vi "MatrixMult (SubVI).vi"(0 "I":fxp<+/-,32,16>, 1 "1,1":fxp<+/-,32,16>, 2 "1, 2":fxp<+/-,32,16>, 3 "1, 3":fxp<+/-,32,16>, 5 "x":fxp<+/-,32,16>, 7 "y":fxp<+/-,32,16>, 9 "3, 1":fxp<+/-,32,16>, 10 "3, 3":fxp<+/-,32,16>, 11 "3, 2":fxp<+/-,32,16>, 12 "2, 1":fxp<+/-,32,16>, 13 "2, 2":fxp<+/-,32,16>, 14 "2, 3":fxp<+/-,32,16>) -> (4 "v1":fxp<+/-,32,16>, 6 "v2":fxp<+/-,32,16>, 8 "v3":fxp<+/-,32,16>)   [LabVIEW 2013]
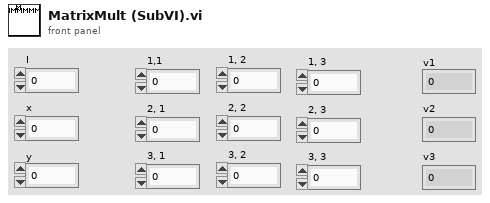
[diagram p1: front panel]
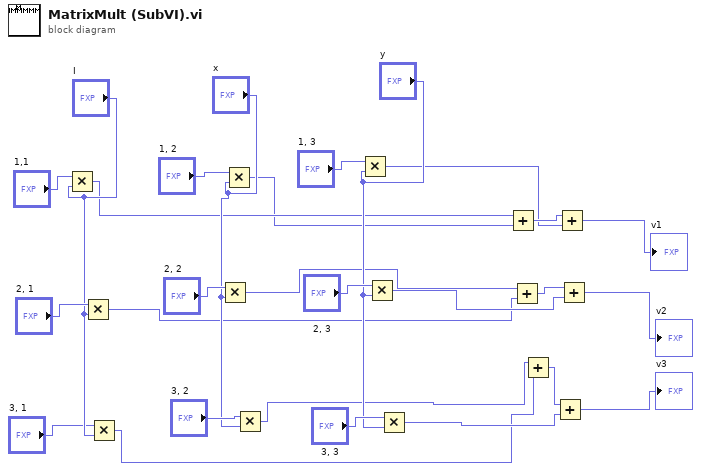
[diagram p0: block diagram]
diagram:
  n1 = Multiply(x="1,1", y="I") -> (x*y=w15:fxp<+/-,32,16>)
  n2 = Multiply(x="2, 1", y="I") -> (x*y=w6:fxp<+/-,32,16>)
  n3 = Multiply(x="3, 1", y="I") -> (x*y=w2:fxp<+/-,32,16>)
  n4 = Multiply(x="2, 2", y="x") -> (x*y=w7:fxp<+/-,32,16>)
  n5 = Multiply(x="1, 2", y="x") -> (x*y=w14:fxp<+/-,32,16>)
  n6 = Multiply(x="3, 2", y="x") -> (x*y=w3:fxp<+/-,32,16>)
  n7 = Multiply(x="1, 3", y="y") -> (x*y=w12:fxp<+/-,32,16>)
  n8 = Multiply(x="2, 3", y="y") -> (x*y=w9:fxp<+/-,32,16>)
  n9 = Multiply(x="3, 3", y="y") -> (x*y=w8:fxp<+/-,32,16>)
  n10 = Add(x=w15, y=w14) -> (x+y=w13:fxp<+/-,32,16>)
  n11 = Add(x=w7, y=w6) -> (x+y=w10:fxp<+/-,32,16>)
  n12 = Add(x=w3, y=w2) -> (x+y=w1:fxp<+/-,32,16>)
  n13 = Add(x=w1, y=w8) -> (x+y=→"v3":fxp<+/-,32,16>)
  n14 = Add(x=w13, y=w12) -> (x+y=→"v1":fxp<+/-,32,16>)
  n15 = Add(x=w10, y=w9) -> (x+y=→"v2":fxp<+/-,32,16>)
